vi "P9P14T_Open_Queue.vi"(8 "error in (no error)":errorcluster) -> (0 "error out":errorcluster, 2 "queue out":refnum<queue>)   [LabVIEW 2019]
uses:
  PPMS/P9P14_Magnet_Control.ctl
  Global/Global Variables/Queues_global.vi
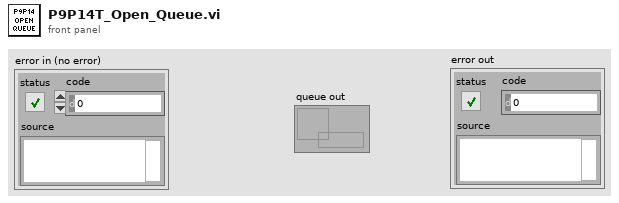
[diagram p1: front panel]
types:
  T1 = typedef "P9P14_Magnet_Control.ctl" = cluster{"Setpoint (Oe)":dbl, "Rate (Oe/min)":dbl, "Set Field":bool, "Go to zero":bool, "Set Persitant/non-pers":bool, "Approach":i32, "Steps":dbl, "Paused Menu":dbl, "B Step start Field":dbl}
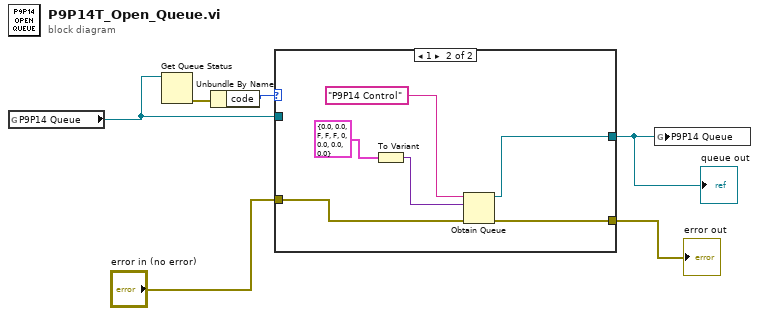
[diagram p0: block diagram]
diagram:
  n1 = global read "Queues_global.vi" "P9P14 Queue"() -> (w6:refnum<queue>)
  n2 = Get Queue Status(queue=w6) -> (error out=w5:errorcluster)  [unwired: 2 in, 7 out]
  n3 = Unbundle By Name(w5) -> ("code"=w4:i32)
  n4 = case shown="1" w4 {
    tunnel: w6 -> [w8 _]
    tunnel: "error in (no error)" -> [w7 w14]
    tunnel: [w7 w13] -> w2
    tunnel: [w8 w9] -> w1
    frame 0, Default {
    }
    frame 1 {
      n5 = To Variant(anything=T1 {"Setpoint (Oe)"=0.0, "Rate (Oe/min)"=0.0, "Set Field"=FALSE, "Go to zero"=FALSE, "Set Persitant/non-pers"=FALSE, "Approach"=0, "Steps"=0.0, "Paused Menu"=0.0, "B Step start Field"=0.0} ("P9/P14-Magnet-Control")) -> (Variant=w11:variant)
      n6 = Obtain Queue(name (unnamed)="P9P14 Control", element data type=w11, error in (no error)=w14) -> (queue out=w9:refnum<queue>, error out=w13:errorcluster)  [unwired: 2 in, 1 out]
    }
  }
  "error out" <- w2
  "queue out" <- w1
  n7 = global write "Queues_global.vi" "P9P14 Queue"(w1) -> ()
